vi "Get Write Data.vi"(8 "Multiplication Factor":dbl=1.0, 9 "Sampling information 2":cluster{"Fs":dbl, "#s":dbl}[](array[cluster])=[{"Fs"=10000.0, "#s"=5000.0}, {"Fs"=10000.0, "#s"=5000.0}], 10 "AO Task":refnum<k21>[](array[refnum])=[""], 11 "OSC Configuration":T1(array[cluster])=[[{"Signal Type"=enum."Sine Wave", "DC"=0.0, "Amplitude"=0.01, "frequency"=2.0, "Phase"=0.0}, {"Signal Type"=enum."Sine Wave", "DC"=0.0, "Amplitude"=0.01, "frequency"=2.0, "Phase"=0.0}], [{"Signal Type"=enum."Sine Wave", "DC"=0.0, "Amplitude"=0.01, "frequency"=2.0, "Phase"=0.0}, {"Signal Type"=enum."Sine Wave", "DC"=0.0, "Amplitude"=0.01, "frequency"=2.0, "Phase"=0.0}]] {"frequency" step=0.001 format="%.3p"; "Amplitude" format="%0.2p"; "DC" min=-0.99 max=0.99 format="%.2p"}) -> (3 "Data":waveform(dbl)[][](array[waveform]))   [LabVIEW 2011, in "Lock-In Variable Channels_2.lvclass"]
uses:
  Variable Channel O.O.P/Lock-In Variable Channels_2.lvclass
  Program Files/National Instruments/LabVIEW 2011/resource/objmgr/daqmx.rc
  <vilib>/measure/NI_MABase.lvlib
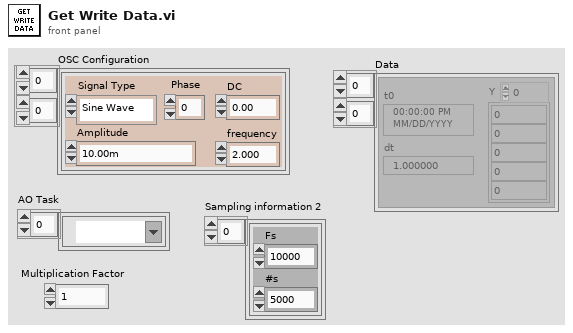
[diagram p1: front panel]
types:
  T1 = cluster{"Signal Type":enum16{"Sine Wave", "Triangle Wave", "Square Wave", "Sawtooth Wave"}, "DC":dbl, "Amplitude":dbl, "frequency":dbl, "Phase":dbl}[][]
  T2 = cluster{"Signal Type":enum16{"Sine Wave", "Triangle Wave", "Square Wave", "Sawtooth Wave"}, "DC":dbl, "Amplitude":dbl, "frequency":dbl, "Phase":dbl}
  T3 = enum16{"Sine Wave", "Triangle Wave", "Square Wave", "Sawtooth Wave"}
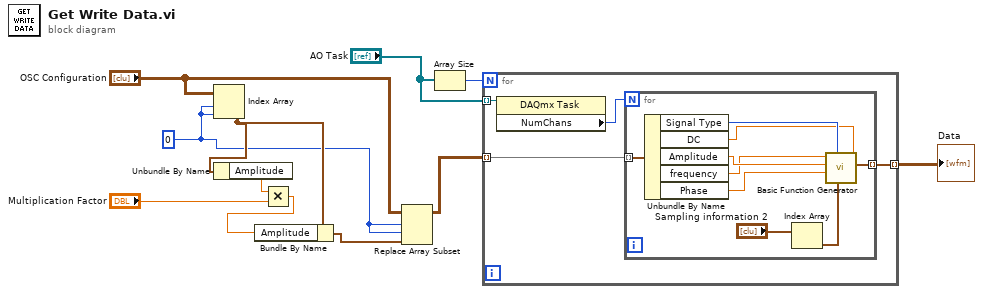
[diagram p0: block diagram]
diagram:
  w7 = 0 ("index")
  n1 = Index Array(array="OSC Configuration", index (row)=w7, index (col)=w7) -> (element=w11:T2)
  n2 = Unbundle By Name(w11) -> ("Amplitude"=w10:dbl)
  n3 = Multiply(x=w10, y="Multiplication Factor") -> (x*y=w9:dbl)
  n4 = Bundle By Name(cluster=w11, "Amplitude"=w9) -> (w8:T2)
  n5 = Replace Array Subset(array="OSC Configuration", new element=w8, index (row)=w7, index (col)=w7) -> (w5:T1)
  n6 = Array Size(array="AO Task") -> (size(s)=w4:i32)
  n7 = for {
    N: w4 -> [_]
    tunnel: [w15] -> w6 mode=indexing
    tunnel: w5 -> [w14] mode=indexing
    tunnel: "AO Task" -> [w12] mode=indexing
    n8 = property class="DAQmx Task"(reference=w12) -> ("NumChans"=w13:u32)  [unwired: 1 in, 2 out]
    n9 = for {
      N: w13 -> [_]
      tunnel: w14 -> [w17] mode=indexing
      tunnel: [w19] -> w15 mode=indexing
      n10 = Unbundle By Name(w17) -> ("Signal Type"=w24:T3, "DC"=w23:dbl, "Amplitude"=w22:dbl, "frequency"=w21:dbl, "Phase"=w20:dbl)
      n11 = Index Array(array="Sampling information 2") -> (element=w18:cluster{"Fs":dbl, "#s":dbl})  [unwired: 1 in]
      n12 = call <vilib>:"Basic Function Generator.vi"("offset"=w23, "sampling info"=w18, "signal type"=w24, "phase"=w20, "amplitude"=w22, "frequency"=w21) -> ("signal out"=w19:waveform(dbl))  [unwired: 3 in, 2 out]
    }
  }
  "Data" <- w6
